vi "DUAL GAUGE_Kammer1.vi"(8 "Fehler (Eingang)":errorcluster) -> (0 "Cluster (Ausgang)":errorcluster, 1 "Pressure FullRange":dbl format="%.3e", 2 "Pressure Baratron":dbl format="%.3e", 3 "COM5 out":refnum<visa-resource-name>, 4 "Status FullRange":i32(ring) items=["data OK", "underrange", "overrange", "sensor error", "sensor off", "no sensor", "ID error"], 5 "Status Baratron":i32(ring) items=["data OK", "underrange", "overrange", "sensor error", "sensor off", "no sensor", "ID error"])   [LabVIEW 2010]
uses:
  Dual Gauge.lvlib
panel:
  in  "Tab Control":enum32{"COM5", "Graph"}(tab)
  out "Cluster (Ausgang) 2":errorcluster caption="Cluster (Ausgang)"
  in  "Fehler (Eingang) 2":errorcluster caption="Fehler (Eingang)"
  out "COM6 out":refnum<visa-resource-name>
  out "Pressure Sensor 4":dbl format="%.3e"
  out "Status Sensor 4":i32(ring) items=["data OK", "underrange", "overrange", "sensor error", "sensor off", "no sensor", "ID error"]
  out "Status Pirani":i32(ring) items=["data OK", "underrange", "overrange", "sensor error", "sensor off", "no sensor", "ID error"]
  out "Pressure Pirani":dbl format="%.3e"
  in  "Offset Control":bool
  out "Pressure":dbl format="%.3e"
  out "Old Offset":dbl format="%.3e"
  out "Current Offset":dbl format="%.3e"
  out "Waveform Chart":T1(graph)
  in  "?":bool
  # "mbar"
  # "mbar"
  # "mbar"
  # "mbar"
  # "mbar"
  # "mbar"
  # "mbar"
  # "mbar"
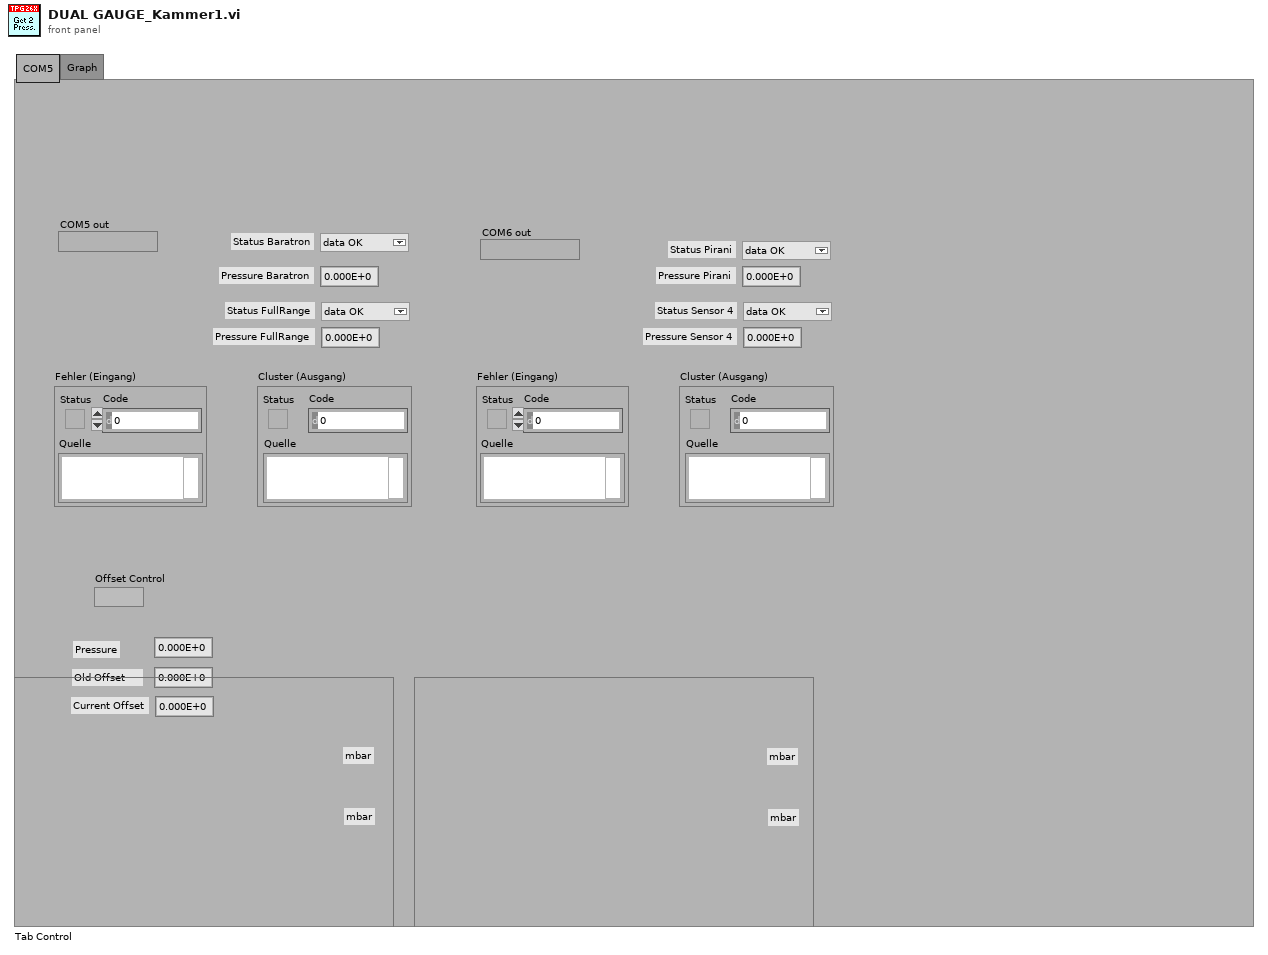
[diagram p1: front panel]
types:
  T1 = cluster{"Eng1 out":dbl, "Eng2 out":dbl, "Eng1 out":dbl, "Eng2 out":dbl}
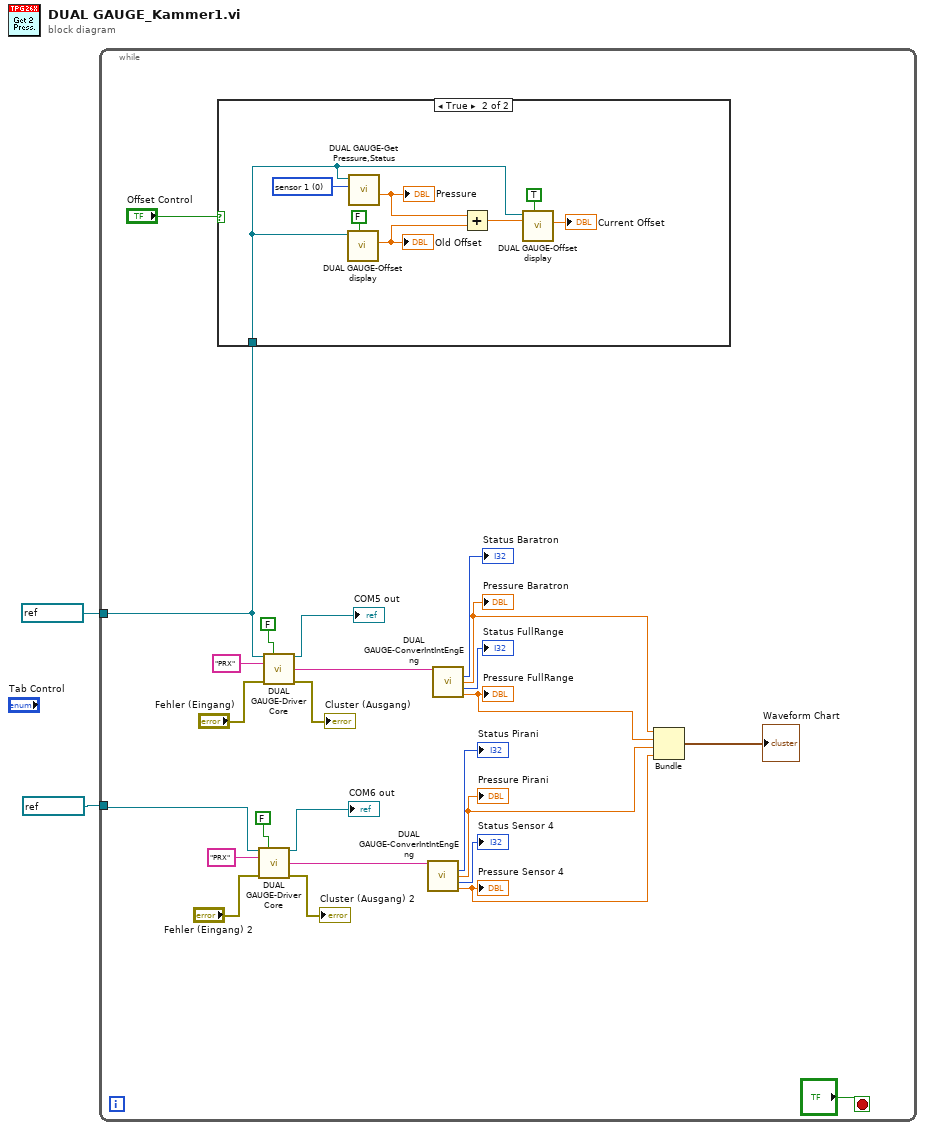
[diagram p0: block diagram]
diagram:
  n1 = while {
    tunnel: refnum<visa-resource-name> "COM5" ("COM5 in") -> [w4]
    tunnel: refnum<visa-resource-name> "COM6" ("COM6 in") -> [w10]
    stop <- "?" stop-if-true
    n2 = case shown="True" "Offset Control" {
      tunnel: w4 -> [_ w35]
      frame False {
      }
      frame True {
        w29 = 0 items=["sensor 1", "sensor 2", "test"] ("Sensor Nr.:")
        n3 = call "DUAL GAUGE-Offset display.vi"("W/R"=FALSE, "Referenz in"=w35) -> ("Sensor 1 Get"=w31:dbl)  [unwired: 6 in, 3 out]
        "Old Offset" <- w31
        n4 = call "DUAL GAUGE-Get Pressure,Status.vi"("Sensor Nr.:"=w29, "Referenz in"=w35) -> ("Pressure"=w32:dbl)  [unwired: 6 in, 3 out]
        "Pressure" <- w32
        n5 = Add(x=w32, y=w31) -> (x+y=w30:dbl)
        n6 = call "DUAL GAUGE-Offset display.vi"("W/R"=TRUE, "Sensor 1 Set"=w30, "Referenz in"=w35) -> ("Sensor 1 Get"=→"Current Offset":dbl)  [unwired: 5 in, 3 out]
      }
    }
    n7 = call "DUAL GAUGE-Driver Core.vi"("Referenz in"=w10, "Write/Read"=FALSE, "Command"="PRX", "Fehler (Eingang)"="Fehler (Eingang) 2") -> ("Referenz out"=→"COM6 out":refnum<visa-resource-name>, "String Out"=w15:string, "Cluster (Ausgang)"=→"Cluster (Ausgang) 2":errorcluster)  [unwired: 9 in]
    n8 = call "DUAL GAUGE-Driver Core.vi"("Referenz in"=w4, "Write/Read"=FALSE, "Command"="PRX", "Fehler (Eingang)"="Fehler (Eingang)") -> ("Referenz out"=→"COM5 out":refnum<visa-resource-name>, "String Out"=w24:string, "Cluster (Ausgang)"=→"Cluster (Ausgang)":errorcluster)  [unwired: 9 in]
    n9 = call "DUAL GAUGE-ConverIntIntEngEng.vi"("String in"=w15) -> ("Integer1 out"=→"Status Pirani":u8, "Eng1 out"=w6:dbl, "Integer2 out"=→"Status Sensor 4":u8, "Eng2 out"=w7:dbl)  [unwired: 11 in]
    "Pressure Pirani" <- w6
    "Pressure Sensor 4" <- w7
    n10 = call "DUAL GAUGE-ConverIntIntEngEng.vi"("String in"=w24) -> ("Integer1 out"=→"Status Baratron":u8, "Eng1 out"=w9:dbl, "Integer2 out"=→"Status FullRange":u8, "Eng2 out"=w8:dbl)  [unwired: 11 in]
    "Pressure Baratron" <- w9
    "Pressure FullRange" <- w8
    n11 = Bundle("Eng1 out"=w9, "Eng2 out"=w8, "Eng1 out"=w6, "Eng2 out"=w7) -> (→"Waveform Chart":T1)  [unwired: 1 in]
  }
